vi "unregisterEvent.vi"(8 "error in (no error)":errorcluster, 10 "name":string, 11 "Event in":refnum<class "Event.lvclass">) -> (0 "error out":errorcluster, 3 "Event out":refnum<class "Event.lvclass">)   [LabVIEW 2011, in "Events.lvlib" / "Event.lvclass"]
uses:
  Event.lvclass
  Event.lvclass/Event.ctl
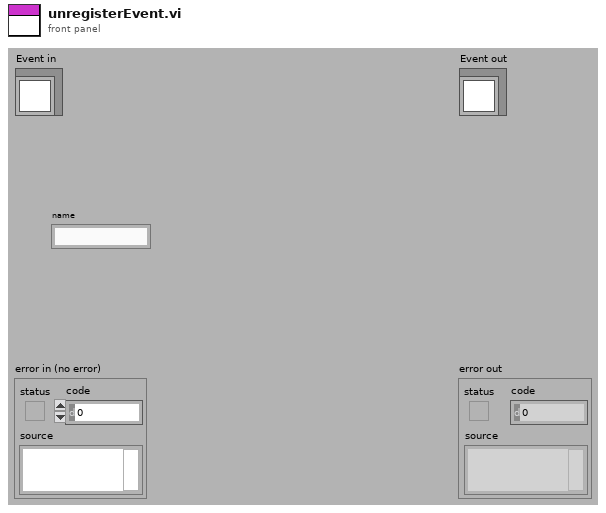
[diagram p1: front panel]
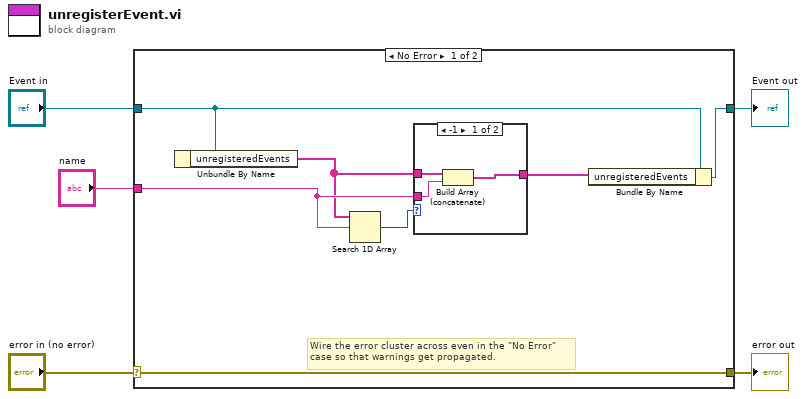
[diagram p0: block diagram]
diagram:
  n1 = case shown="No Error" "error in (no error)" {
    selector: "error in (no error)" -> [w12 w18]
    tunnel: [w12 w18] -> w4
    tunnel: [w6 w17] -> w2
    tunnel: "Event in" -> [w7 w17]
    tunnel: "name" -> [w10 _]
    frame No Error {
      # "Wire the error cluster across even in the \"No Error\"\ncase so that warnings get propagated."
      n2 = Unbundle By Name(w7) -> ("unregisteredEvents"=w9:string[])
      n3 = Search 1D Array(1D array=w9, element=w10) -> (index of element=w11:i32)  [unwired: 1 in]
      n4 = case shown="-1" w11 {
        tunnel: w10 -> [w15 _]
        tunnel: w9 -> [w14 w16]
        tunnel: [w13 w16] -> w8
        frame -1 {
          n5 = Build Array (concatenate)(w14, w15) -> (w13:string[])
        }
        frame Default {
        }
      }
      n6 = Bundle By Name(cluster=w7, "unregisteredEvents"=w8) -> (w6:refnum<class "Event.lvclass">)
    }
    frame Error {
    }
  }
  "error out" <- w4
  "Event out" <- w2
